vi "UTILITY Error Bool Add Message.vi"(5 "Error?":bool, 7 "Message":string, 11 "Error In":errorcluster) -> (15 "Error Out":errorcluster)   [LabVIEW 2016]
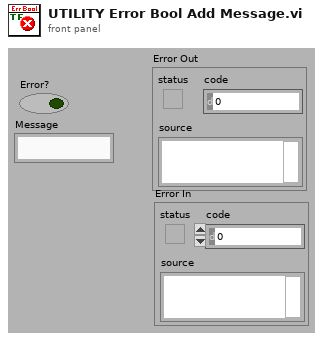
[diagram p1: front panel]
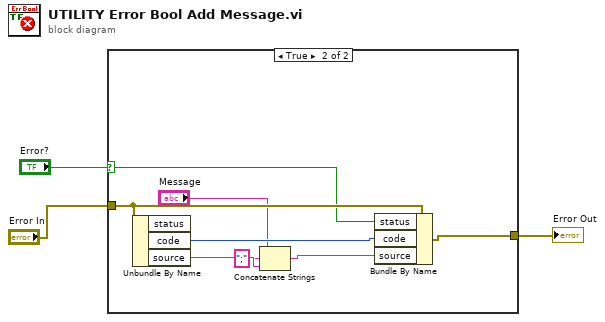
[diagram p0: block diagram]
diagram:
  n1 = case shown="True" "Error?" {
    selector: "Error?" -> [_ w9]
    tunnel: "Error In" -> [w4 w12]
    tunnel: [w4 w5] -> w1
    frame False {
    }
    frame True {
      n2 = Unbundle By Name(w12) -> ("code"=w10:i32, "source"=w8:string)  [unwired: 1 out]
      n3 = Concatenate Strings("Message", ";" ("string"), w8) -> (w11:string)
      n4 = Bundle By Name(cluster=w12, "status"=w9, "code"=w10, "source"=w11) -> (w5:errorcluster)
    }
  }
  "Error Out" <- w1
